vi "CRYCheck Calibration Step.vi"(11 "Step No":i32=3) -> (2 "CalibrationStepNo Out":i32, 3 "Is Calibration?":bool)   [LabVIEW 2013]
uses:
  CRYProject Editor Global.vi
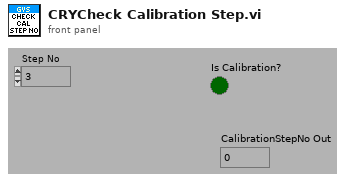
[diagram p1: front panel]
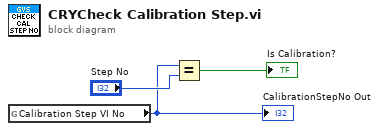
[diagram p0: block diagram]
diagram:
  n1 = global read "CRYProject Editor Global.vi" "Calibration Step VI No"() -> (w1:i32)
  "CalibrationStepNo Out" <- w1
  n2 = Equal?(x=w1, y="Step No") -> (x = y?=→"Is Calibration?":bool)
